vi "scriptRunner.vi"(8 "error in (no error)":errorcluster, 9 "script":string, 10 "matlabScript":string, 11 "MatlabScripts in":refnum<class "MatlabScripts.lvclass">) -> (0 "error out":errorcluster, 3 "MatlabScripts out":refnum<class "MatlabScripts.lvclass">)   [LabVIEW 2011, in "Views.lvlib" / "ExperimentControl.lvlib" / "MatlabScripts.lvclass"]
uses:
  MatlabScripts.lvclass
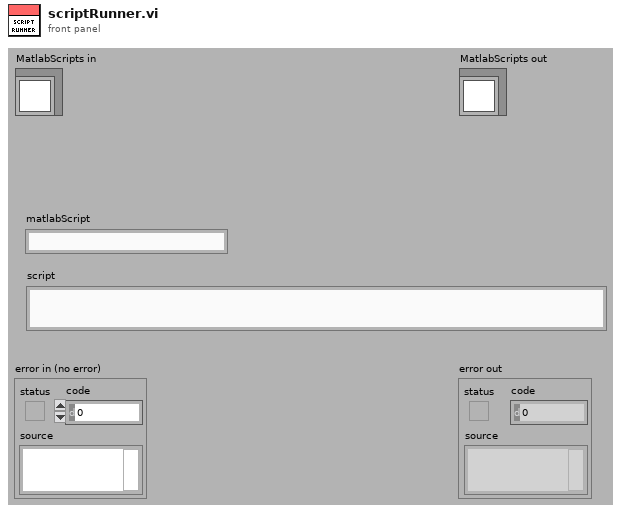
[diagram p1: front panel]
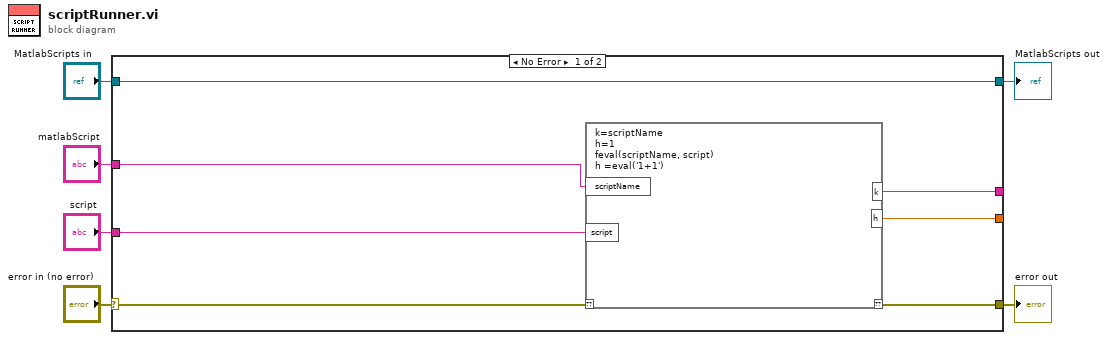
[diagram p0: block diagram]
diagram:
  n1 = case shown="No Error" "error in (no error)" {
    selector: "error in (no error)" -> [w12 w15]
    tunnel: [w11 w15] -> w5
    tunnel: [w13 w14] -> w3
    tunnel: "MatlabScripts in" -> [w13 w14]
    tunnel: "matlabScript" -> [w10 _]
    tunnel: "script" -> [w7 _]
    tunnel: [w9 _] -> _
    tunnel: [w8 _] -> _
    frame No Error {
      n2 = script code="k=scriptName\nh=1\nfeval(scriptName, script)\nh =eval('1+1')"("??"=w12, "scriptName"=w10, "script"=w7) -> ("??"=w11:errorcluster, "k"=w9:string, "h"=w8:dbl)
    }
    frame Error {
    }
  }
  "error out" <- w5
  "MatlabScripts out" <- w3
